vi "Transmit Messages with Rate-based Schedule.vi"() -> ()   [LabVIEW 2019]
doc: "This program opens the specified card, builds a transmit schedule \nusing transmit interval information in the channel configuration file,\nand then transmits the messages with changing data."
uses:
  <instrlib>/BTICardLib/Private/Initialize By Card Number and Core Number.vi
  <instrlib>/BTICardLib/Private/Configure Core From XML.vi
  <instrlib>/BTI429Lib/Private/Tx/Configure/Configure Tx Channel From XML.vi
  <instrlib>/BTI429Lib/Private/Core/Action-Status/Start Channel.vi
  <instrlib>/BTI429Lib/Private/Utility/Get BNR Mantissa.vi
  <instrlib>/BTI429Lib/Private/Utility/Set BNR Mantissa.vi
  <instrlib>/BTI429Lib/Private/Core/Action-Status/Stop Channel.vi
  <instrlib>/BTICardLib/BTICardLV.lvlib
  <instrlib>/BTI429Lib/BTI429LV.lvlib
panel:
  out "core number":i32
  out "channel number":i32
  in  "Core Configuration XML file name":string="Core Config.xml"
  in  "Channel Configuration XML file name":string="Channel Config.xml"
  out "error out":errorcluster
  in  "stop":bool
  out "Data 1":u32 format="%.0x"
  out "Data 2":u32 format="%.0x"
  out "Data 3":u32 format="%.0x"
  in  "Card Number":i32
  # "ARINC 429: Transmit Messages with Rate-based Schedule"
  # "©2016 Astronics Ballard Technology"
  # "This program opens the specified card, builds a transmit schedule \nusing transmit interval information in the channel configuration file,\nand then transmits the messages with changing data."
  # "Always Stop the card\nand Close the card when\ndone. Otherwise, the hardware\ncontinues to operate."
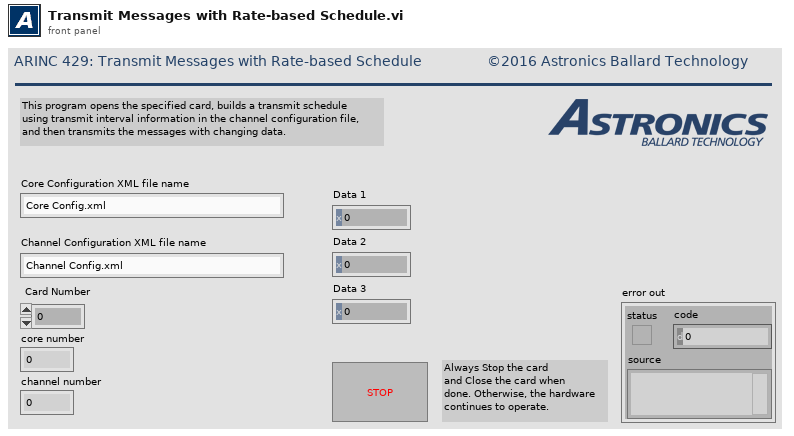
[diagram p1: front panel]
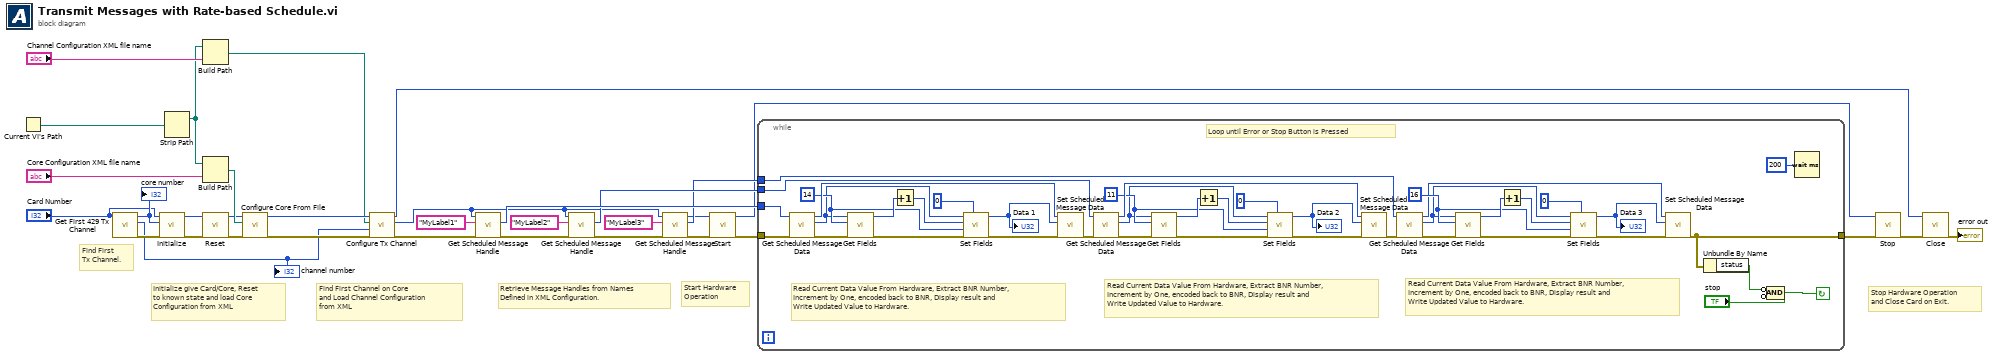
[diagram p0: block diagram]
diagram:
  # "Find First\nTx Channel."
  # "Stop Hardware Operation\nand Close Card on Exit."
  # "Start Hardware\nOperation"
  # "Retrieve Message Handles from Names\nDefined in XML Configuration."
  # "Find First Channel on Core\nand Load Channel Configuration\nfrom XML"
  # "Initialize give Card/Core, Reset\nto known state and load Core\nConfiguration from XML"
  n1 = Current VI's Path() -> (path=w14:path)
  n2 = call "Get First 429 Tx Channel.vi"("Card Number"="Card Number") -> ("error out"=w2:errorcluster, "Channel Number"=w1:i32, "Core Number"=w4:i32)  [unwired: 8 in]
  "channel number" <- w1
  "core number" <- w4
  n3 = call-poly <instrlib>:"Initialize.vi"("error in (no error)"=w2, "core number"=w4, "card number"="Card Number") -> ("error out"=w7:errorcluster, "core handle out"=w8:u64)  [unwired: 7 in]
  n4 = Strip Path(path=w14) -> (stripped path=w11:path)  [unwired: 1 out]
  n5 = Build Path(base path=w11, name or relative path="Channel Configuration XML file name") -> (appended path=w13:path)
  n6 = Build Path(base path=w11, name or relative path="Core Configuration XML file name") -> (appended path=w9:path)
  n7 = call <instrlib>:"Reset.vi"("error in (no error)"=w7, "core handle in"=w8) -> ("error out"=w5:errorcluster, "core handle out"=w6:u64)  [unwired: 8 in]
  n8 = call-poly <instrlib>:"Configure Core From File.vi"("error in (no error)"=w5, "configuration file path"=w9, "core handle in"=w6) -> ("error out"=w20:errorcluster, "core handle out"=w19:u64)  [unwired: 7 in]
  n9 = call-poly <instrlib>:"Configure Tx Channel.vi"("error in (no error)"=w20, "channel number in"=w1, "configuration file path"=w13, "core handle in"=w19) -> ("error out"=w34:errorcluster, "channel handle out"=w22:u64, "core handle out"=w21:u64)  [unwired: 5 in]
  n10 = call <instrlib>:"Get Scheduled Message Handle.vi"("error in (no error)"=w34, "message name"="MyLabel1" ("msgname"), "channel handle in"=w22) -> ("error out"=w29:errorcluster, "message handle out"=w32:u64)  [unwired: 6 in, 1 out]
  n11 = call <instrlib>:"Get Scheduled Message Handle.vi"("error in (no error)"=w29, "message name"="MyLabel2" ("msgname"), "channel handle in"=w22) -> ("error out"=w28:errorcluster, "message handle out"=w31:u64)  [unwired: 6 in, 1 out]
  n12 = call <instrlib>:"Get Scheduled Message Handle.vi"("error in (no error)"=w28, "message name"="MyLabel3" ("msgname"), "channel handle in"=w22) -> ("error out"=w27:errorcluster, "message handle out"=w30:u64, "channel handle out"=w16:u64)  [unwired: 6 in]
  n13 = call-poly <instrlib>:"Start.vi"("error in (no error)"=w27, "channel handle in"=w16) -> ("error out"=w33:errorcluster, "channel handle out"=w18:u64)  [unwired: 8 in]
  n14 = while {
    tunnel: [w44] -> w17
    tunnel: w30 -> [w47]
    tunnel: w31 -> [w58]
    tunnel: w33 -> [w67]
    tunnel: w32 -> [w57]
    stop <- w73 continue-if-true
    w41 = u16 16
    w42 = u16 11
    w43 = u16 14
    # "Read Current Data Value From Hardware, Extract BNR Number,\nIncrement by One, encoded back to BNR, Display result and\nWrite Updated Value to Hardware."
    # "Read Current Data Value From Hardware, Extract BNR Number,\nIncrement by One, encoded back to BNR, Display result and\nWrite Updated Value to Hardware."
    # "Read Current Data Value From Hardware, Extract BNR Number,\nIncrement by One, encoded back to BNR, Display result and\nWrite Updated Value to Hardware."
    # "Loop until Error or Stop Button is Pressed"
    n15 = call <instrlib>:"Get Scheduled Message Data.vi"("error in (no error)"=w67, "message handle in"=w57) -> ("error out"=w72:errorcluster, "value"=w36:u32, "message handle out"=w65:u64)  [unwired: 7 in]
    n16 = call-poly <instrlib>:"Get Fields.vi"("error in (no error)"=w72, "significant digits"=w43, "message"=w36) -> ("error out"=w71:errorcluster, "mantissa out"=w69:u32)  [unwired: 7 in]
    n17 = Increment(x=w69) -> (x+1=w68:u32)
    n18 = call-poly <instrlib>:"Set Fields.vi"("twos"=u16 0, "error in (no error)"=w71, "significant bits"=w43, "value"=w68, "message"=w36) -> ("error out"=w70:errorcluster, "message out"=w37:u32)  [unwired: 5 in]
    "Data 1" <- w37
    n19 = call <instrlib>:"Set Scheduled Message Data.vi"("error in (no error)"=w70, "value"=w37, "message handle in"=w65) -> ("error out"=w54:errorcluster)  [unwired: 7 in, 1 out]
    n20 = call <instrlib>:"Get Scheduled Message Data.vi"("error in (no error)"=w54, "message handle in"=w58) -> ("error out"=w64:errorcluster, "value"=w38:u32, "message handle out"=w59:u64)  [unwired: 7 in]
    n21 = call-poly <instrlib>:"Get Fields.vi"("error in (no error)"=w64, "significant digits"=w42, "message"=w38) -> ("error out"=w63:errorcluster, "mantissa out"=w61:u32)  [unwired: 7 in]
    n22 = Increment(x=w61) -> (x+1=w60:u32)
    n23 = call-poly <instrlib>:"Set Fields.vi"("twos"=u16 0, "error in (no error)"=w63, "significant bits"=w42, "value"=w60, "message"=w38) -> ("error out"=w62:errorcluster, "message out"=w55:u32)  [unwired: 5 in]
    "Data 2" <- w55
    n24 = call <instrlib>:"Set Scheduled Message Data.vi"("error in (no error)"=w62, "value"=w55, "message handle in"=w59) -> ("error out"=w48:errorcluster)  [unwired: 7 in, 1 out]
    n25 = call <instrlib>:"Get Scheduled Message Data.vi"("error in (no error)"=w48, "message handle in"=w47) -> ("error out"=w53:errorcluster, "value"=w39:u32, "message handle out"=w40:u64)  [unwired: 7 in]
    n26 = call-poly <instrlib>:"Get Fields.vi"("error in (no error)"=w53, "significant digits"=w41, "message"=w39) -> ("error out"=w52:errorcluster, "mantissa out"=w50:u32)  [unwired: 7 in]
    n27 = Increment(x=w50) -> (x+1=w49:u32)
    n28 = call-poly <instrlib>:"Set Fields.vi"("twos"=u16 0, "error in (no error)"=w52, "significant bits"=w41, "value"=w49, "message"=w39) -> ("error out"=w51:errorcluster, "message out"=w46:u32)  [unwired: 5 in]
    "Data 3" <- w46
    n29 = call <instrlib>:"Set Scheduled Message Data.vi"("error in (no error)"=w51, "value"=w46, "message handle in"=w40) -> ("error out"=w44:errorcluster)  [unwired: 7 in, 1 out]
    n30 = Unbundle By Name(w44) -> ("status"=w74:bool)
    n31 = Compound Arithmetic op=AND(invert w74, invert "stop") -> (w73:bool)
    n32 = Wait (ms)(milliseconds to wait=u32 200) -> ()  [unwired: 1 out]
  }
  n33 = call-poly <instrlib>:"Stop.vi"("error in (no error)"=w17, "channel handle in"=w18) -> ("error out"=w15:errorcluster)  [unwired: 8 in, 1 out]
  n34 = call <instrlib>:"Close.vi"("error in (no error)"=w15, "core handle in"=w21) -> ("error out"=→"error out":errorcluster)  [unwired: 8 in, 1 out]
